vi "Get State.vi"(6 "Controller name":string, 8 "error in (no error)":errorcluster, 11 "Pulse Controller in":refnum<class "Pulse Recorder Actor.lvclass">) -> (0 "error out":errorcluster, 1 "Result ready":bool, 2 "Armed":bool, 3 "Pulse Controller out":refnum<class "Pulse Recorder Actor.lvclass">, 4 "Check again":bool)   [LabVIEW 2021, in "Pulse Recorder Actor.lvclass"]
uses:
  Pulse Recorder Actor.lvclass
  Pulse Recorder Actor.lvclass/Pulse Recorder Actor.ctl
  Instrument Actor/Instrument Actor.lvclass
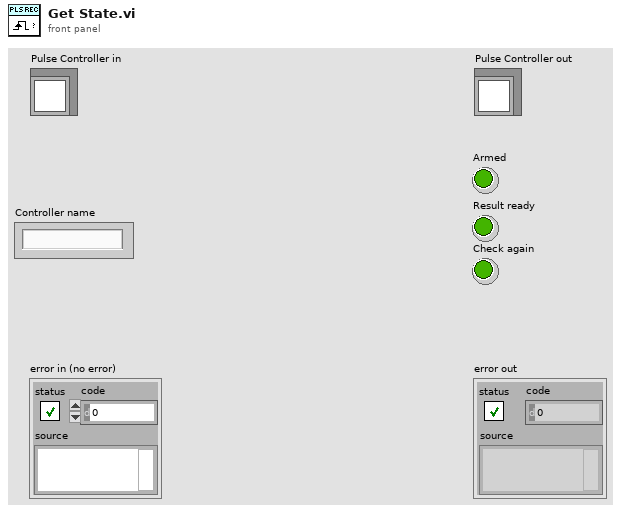
[diagram p1: front panel]
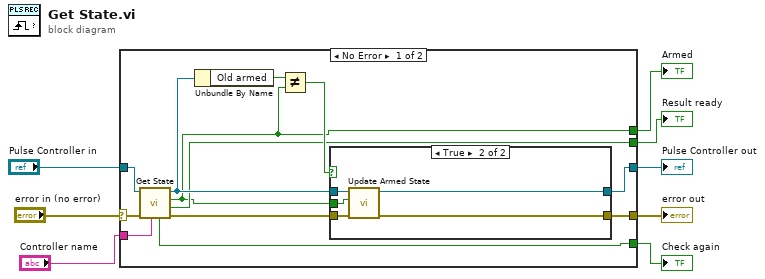
[diagram p0: block diagram]
diagram:
  n1 = case shown="No Error" "error in (no error)" {
    selector: "error in (no error)" -> [w17 w29]
    tunnel: [w18 w29] -> w7
    tunnel: [w14 w28] -> w5
    tunnel: "Pulse Controller in" -> [w16 w28]
    tunnel: [w12 _] -> w4
    tunnel: [w11 _] -> w3
    tunnel: [w10 _] -> w2
    tunnel: "Controller name" -> [w9 _]
    frame No Error {
      n2 = call-parent "Get State.vi"("Controller name"=w9, "error in (no error)"=w17, "Instrument Actor in"=w16) -> ("error out"=w13:errorcluster, "Result ready"=w11:bool, "Armed"=w10:bool, "Instrument Actor out"=w15:refnum<class "Pulse Recorder Actor.lvclass">, "Check again"=w12:bool)  [unwired: 4 in]
      n3 = Unbundle By Name(w15) -> ("Old armed"=w20:bool)
      n4 = Not Equal?(x=w20, y=w10) -> (x != y?=w19:bool)
      n5 = case shown="True" w19 {
        tunnel: w15 -> [w21 w27]
        tunnel: w13 -> [w22 w26]
        tunnel: [w22 w25] -> w18
        tunnel: w10 -> [_ w23]
        tunnel: [w21 w24] -> w14
        frame False {
        }
        frame True {
          n6 = call-dynamic "Update Armed State.vi"("error in (no error)"=w26, "Armed"=w23, "Pulse Recorder in"=w27) -> ("error out"=w25:errorcluster, "Pulse Recorder out"=w24:refnum<class "Pulse Recorder Actor.lvclass">)  [unwired: 7 in]
        }
      }
    }
    frame Error {
    }
  }
  "error out" <- w7
  "Pulse Controller out" <- w5
  "Check again" <- w4
  "Result ready" <- w3
  "Armed" <- w2
